vi "Merge Error.vi"(10 "Error":errorcluster, 11 "jettl Msg Merge Error in":refnum<class "jettl Msg Merge Error.lvclass">) -> (3 "jettl Msg Merge Error out":refnum<class "jettl Msg Merge Error.lvclass">)   [LabVIEW 2021, in "jettl Msg Merge Error.lvlib" / "jettl Msg Merge Error.lvclass"]
uses:
  jettl Msg Merge Error.lvclass
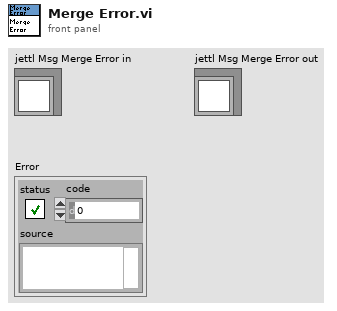
[diagram p1: front panel]
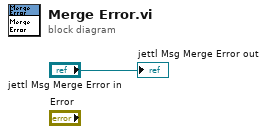
[diagram p0: block diagram]
diagram:
  "jettl Msg Merge Error out" <- "jettl Msg Merge Error in"
